vi "getConnectionPoint.vi"(0 "reference":refnum<class "AbstractNode.lvclass">, 1 "direction":refnum<class "Direction.lvclass">, 5 "error in (no error)":errorcluster) -> (14 "reference out":refnum<class "AbstractNode.lvclass">, 15 "point2D":T1 {"y" format="%.2f"; "x" format="%.2f"}, 19 "error out":errorcluster)   [LabVIEW 2016, in "AbstractNode.lvclass"]
uses:
  <resource>/Framework/Providers/Open_GDS/UML/AbstractNode_class/AbstractNode.lvclass
  <resource>/Framework/Providers/Open_GDS/UML/Direction_class/Direction.lvclass
  <resource>/Framework/Providers/Open_GDS/UML/General/Point/Point Point2D.ctl
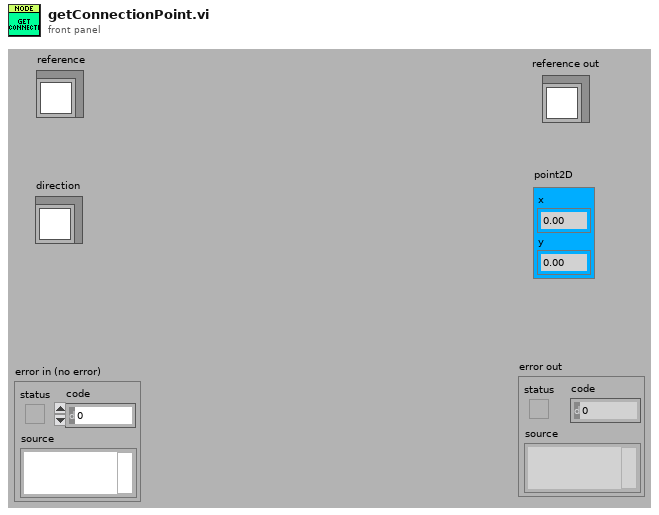
[diagram p1: front panel]
types:
  T1 = typedef "Point Point2D.ctl" = cluster{"x":dbl, "y":dbl}
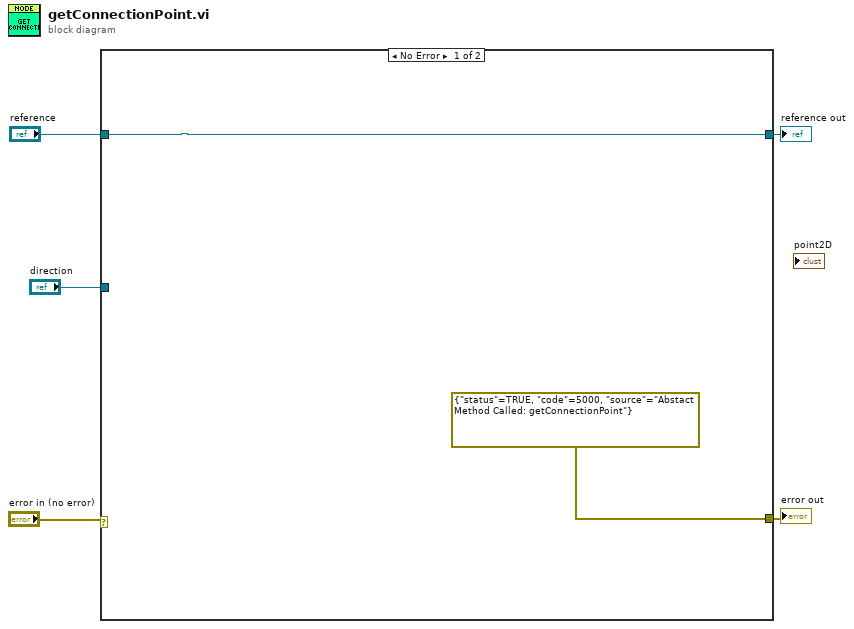
[diagram p0: block diagram]
diagram:
  n1 = case shown="No Error" "error in (no error)" {
    selector: "error in (no error)" -> [_ w8]
    tunnel: "reference" -> [w7 w9]
    tunnel: [errorcluster {"status"=TRUE, "code"=5000, "source"="Abstact Method Called: getConnectionPoint"} ("error out") w8] -> w4
    tunnel: [w7 w9] -> w3
    tunnel: "direction" -> [_ _]
    frame No Error {
    }
    frame Error {
    }
  }
  "reference out" <- w3
  "error out" <- w4
